vi "Stakeholder id assign.vi"() -> ()   [LabVIEW 2017]
uses:
  <vilib>/Utility/miscctls.llb/LVRowAndColumnTypeDef.ctl
  <vilib>/Utility/miscctls.llb/LVBoundsTypeDef.ctl
  <vilib>/addons/database/Connection.llb/DB Tools Open Connec (Path).vi
  <vilib>/addons/database/NI_Database_API.lvlib
panel:
  in  "Cancel Button - Archive":bool
  in  "Update Button":bool
  in  "Select ID":string(combo)
  out "error out":errorcluster
  in  "error in (no error)":errorcluster
  in  "Enter Stakeholder's Name":string
  out "Table":string[][](table)
  # "Stakeholder ID Assign"
  # "Designed And Developed By - Infinity Automation Systems Pvt. Ltd."
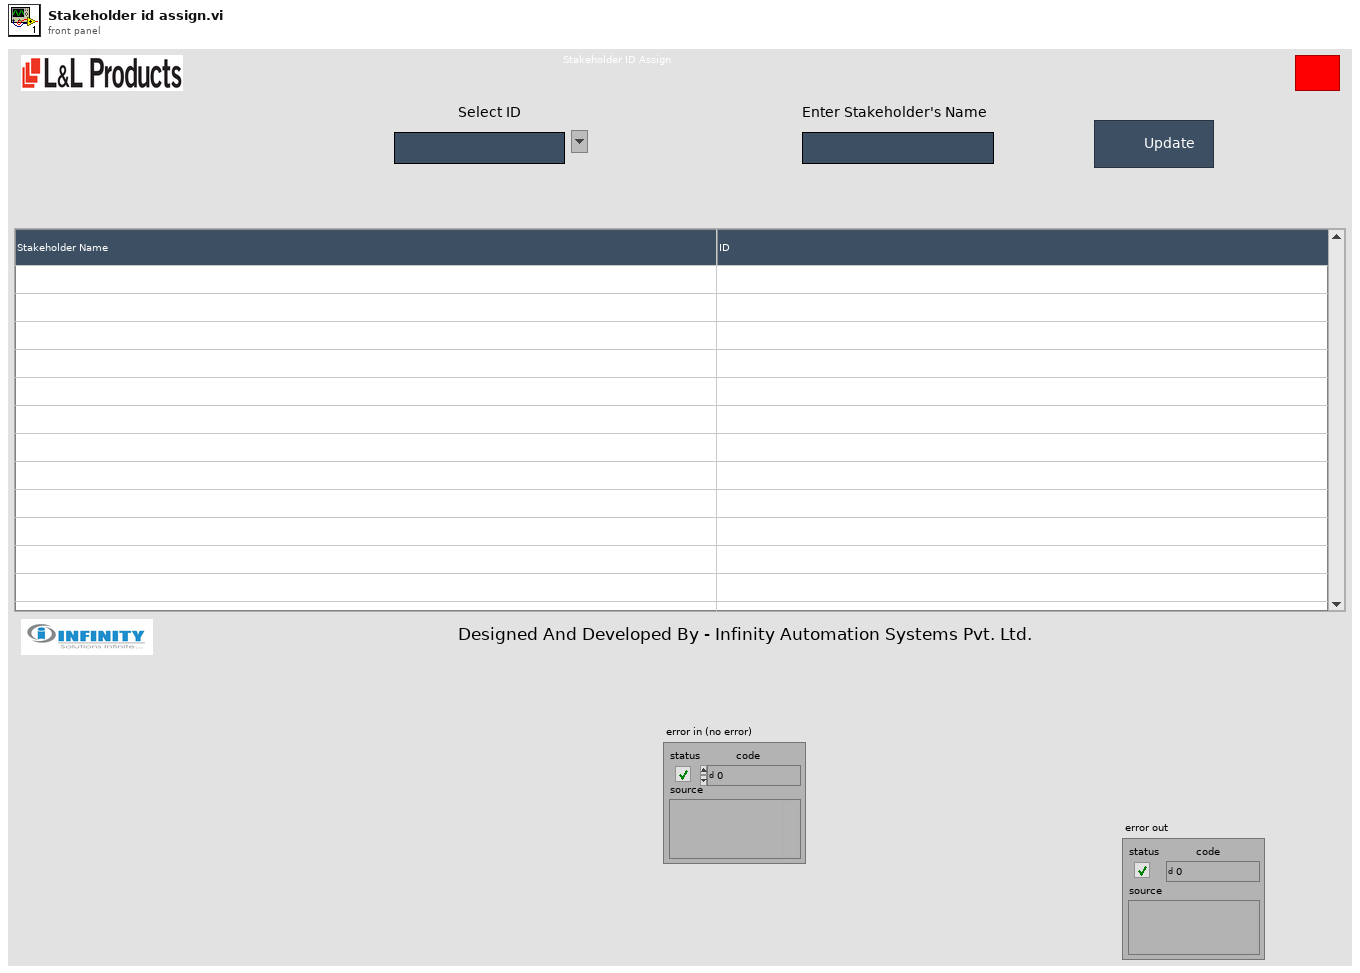
[diagram p1: front panel]
types:
  T1 = typedef "LVBoundsTypeDef.ctl" = cluster{"Width":u32, "Height":u32}
  T2 = typedef "LVRowAndColumnTypeDef.ctl" = cluster{"Row":i32, "Column":i32}
  T3 = typedef "NI_Database_API.lvlib/Conn ObjectReference.ctl" = refnum<k1>
  T4 = enum32{"invalid app kind", "Development System", "Run Time System", "Student Edition", "Embedded LabVIEW", "Evaluation", "Custom"}
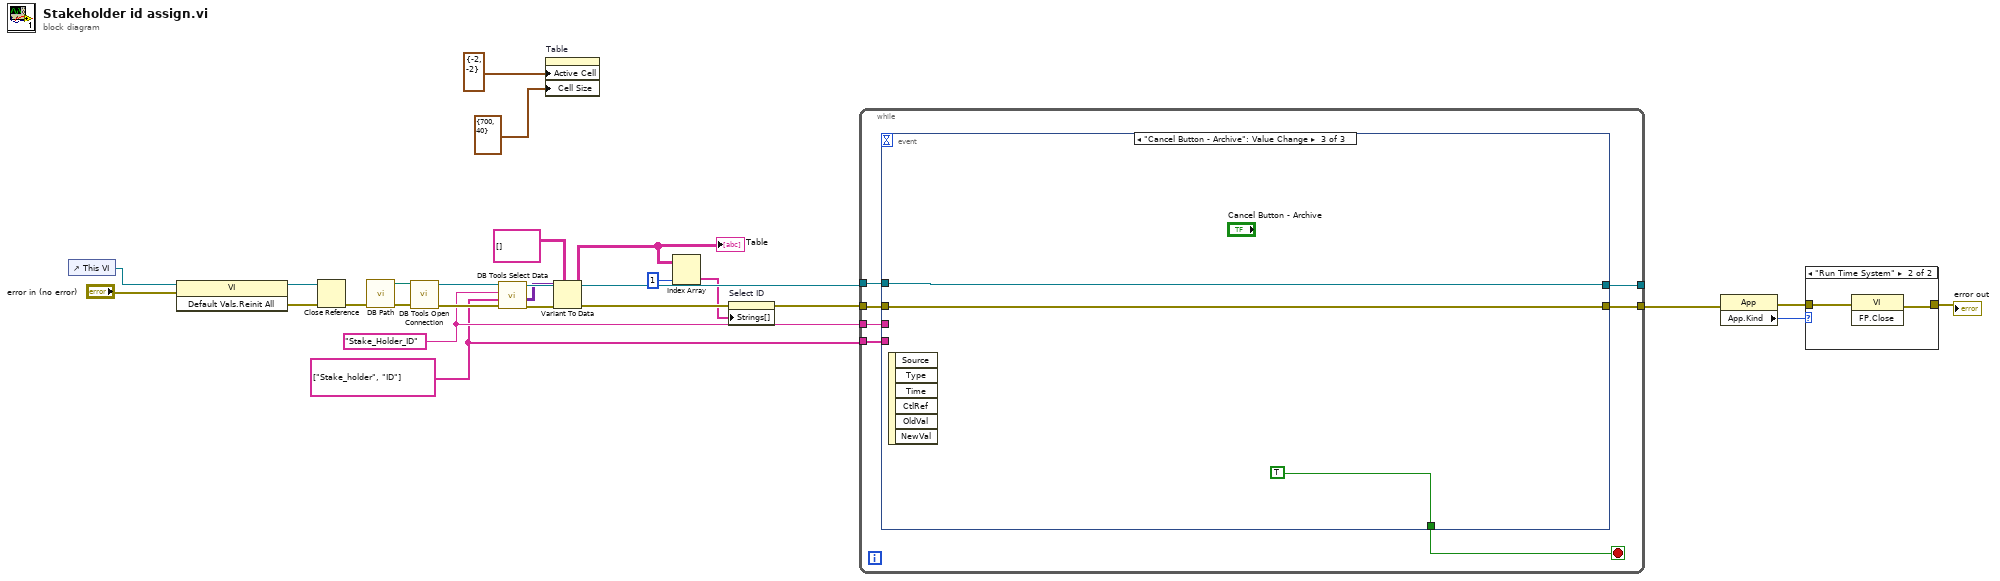
[diagram p0: block diagram]
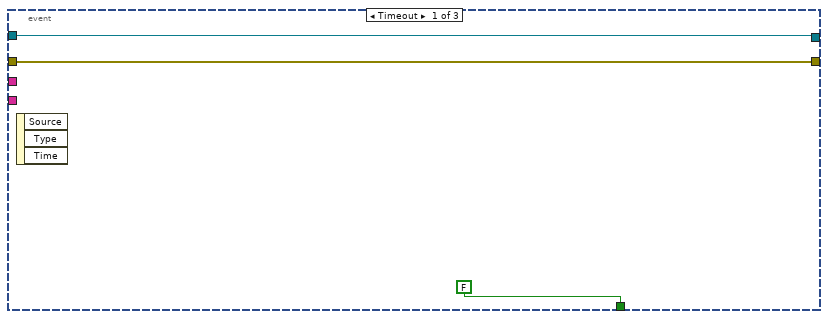
[diagram p3: hidden frame]
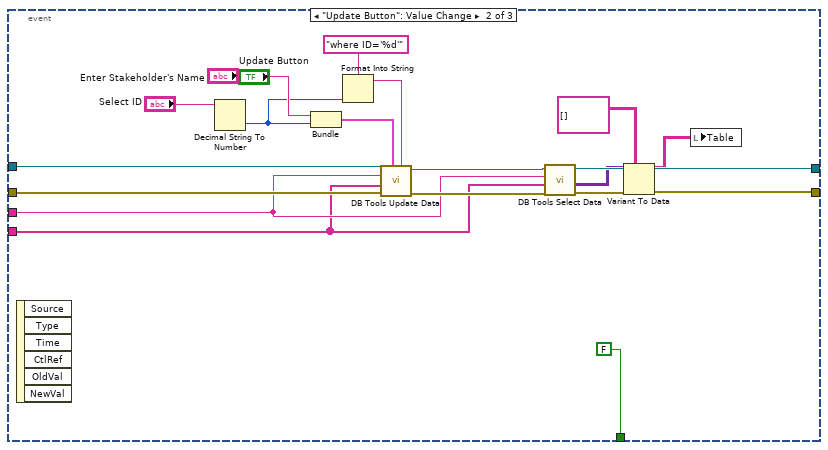
[diagram p4: hidden frame]
diagram:
  w6 = string[] ["Stake_holder", "ID"]
  w11 = "Stake_Holder_ID" ("table")
  n1 = control-ref of="This VI"() -> (w24:refnum<vi>)
  n2 = invoke class="VI" method="Default Vals.Reinit All"(reference=w24, error in="error in (no error)") -> (reference out=w21:refnum<vi>, error out=w22:errorcluster)  [unwired: 1 in, 1 out]
  n3 = Close Reference(reference=w21, error in (no error)=w22) -> (error out=w17:errorcluster)
  n4 = call "DB Path.vi"("error in"=w17) -> ("error out"=w16:errorcluster, "DB Path"=w15:path)  [unwired: 9 in]
  n5 = call-poly <vilib>:"DB Tools Open Connection.vi"("error in (no error)"=w16, "connection information"=w15) -> ("error out"=w14:errorcluster, "connection reference"=w13:T3)  [unwired: 6 in]
  n6 = call <vilib>:"DB Tools Select Data.vi"("error in (no error)"=w14, "columns"=w6, "table"=w11, "connection reference"=w13) -> ("error out"=w10:errorcluster, "data"=w9:variant[][], "connection reference out"=w12:T3)  [unwired: 2 in]
  n7 = property on="Table" class="Tbl (strict)"("Active Cell"=T2 {"Row"=-2, "Column"=-2} ("Active Cell:Active Cell"), "Cell Size"=T1 {"Width"=700, "Height"=40} ("Active Cell:Cell Size")) -> ()  [unwired: 2 in, 2 out]
  n8 = Variant To Data(error in=w10, type=string[][] [], Variant=w9) -> (data=w5:string[][], error out=w3:errorcluster)
  "Table" <- w5
  n9 = Index Array(array=w5, index (col)=1 ("disabled index (col)")) -> (element=w1:string[])  [unwired: 1 in]
  n10 = property on="Select ID" class="CmbBox"(error in=w3, "Strings[]"=w1) -> (error out=w2:errorcluster)  [unwired: 1 in, 1 out]
  n11 = while {
    tunnel: w2 -> [w33]
    tunnel: w12 -> [w32]
    tunnel: [w31] -> w7
    tunnel: [w30] -> _
    tunnel: w6 -> [w29]
    tunnel: w11 -> [w28]
    stop <- w27 stop-if-true
    n12 = event shown="[2] \"Cancel Button - Archive\": Value Change" {
      selector: _ -> [_ _ _]
      dyn-events: _ -> [_ _ _]
      timeout: _ -> [_ _ _]
      tunnel: w33 -> [w35 w46 w57]
      tunnel: w32 -> [w34 w41 w58]
      tunnel: [w35 w52 w57] -> w31
      tunnel: [w34 w54 w58] -> w30
      tunnel: w29 -> [_ w42 _]
      tunnel: w28 -> [_ w43 _]
      tunnel: [FALSE FALSE TRUE] -> w27
      event Timeout {
        n13 = event-data() -> ()  [unwired: 1 in, 3 out]
      }
      event "Update Button": Value Change {
        n14 = event-data() -> ()  [unwired: 1 in, 6 out]
        n15 = Decimal String To Number(string="Select ID") -> (number=w39:i32)  [unwired: 2 in, 1 out]
        n16 = Bundle("Enter Stakeholder's Name"="Enter Stakeholder's Name", w39) -> (w44:cluster{"Enter Stakeholder's Name":string, i32})  [unwired: 1 in]
        n17 = Format Into String(format string="where ID='%d'", w39) -> (resulting string=w37:string)  [unwired: 2 in, 1 out]
        n18 = call <vilib>:"DB Tools Update Data.vi"("condition"=w37, "data"=w44, "error in (no error)"=w46, "columns"=w42, "table"=w43, "connection reference"=w41) -> ("error out"=w45:errorcluster, "connection reference out"=w40:T3)  [unwired: 4 in]
        n19 = call <vilib>:"DB Tools Select Data.vi"("error in (no error)"=w45, "columns"=w42, "table"=w43, "connection reference"=w40) -> ("error out"=w53:errorcluster, "data"=w50:variant[][], "connection reference out"=w54:T3)  [unwired: 2 in]
        n20 = Variant To Data(error in=w53, type=string[][] [], Variant=w50) -> (data=w49:string[][], error out=w52:errorcluster)
        n21 = local write "Table"(w49) -> ()
      }
      event "Cancel Button - Archive": Value Change {
        n22 = event-data() -> ()  [unwired: 1 in, 6 out]
      }
    }
  }
  n23 = property class="App"(error in=w7) -> (error out=w19:errorcluster, "App.Kind"=w20:T4)  [unwired: 1 in, 1 out]
  n24 = case shown="\"Run Time System\"" w20 {
    tunnel: w19 -> [w59 w61]
    tunnel: [w59 w60] -> w18
    frame Default {
    }
    frame "Run Time System" {
      n25 = invoke class="VI" method="FP.Close"(error in=w61) -> (error out=w60:errorcluster)  [unwired: 2 in, 2 out]
    }
  }
  "error out" <- w18
